vi "DG5252_VI.vi"(5 "DC Offset (0.00 V)":dbl, 6 "Frequency (1000 Hz)":dbl=1000.0, 7 "Unit (0: Vpp)":u16(ring) items=["Vpp", "Vrms", "dB"], 8 "Amplitude (1)":dbl=1.0, 9 "Waveform Function":u16(ring) items=["Sine", "Square", "Ramp", "Pulse", "Noise", "DC", "User"], 10 "Channel Selection":u16(ring) items=["Channel 1", "Channel 2"], 11 "VISA resource name":refnum<visa-resource-name>) -> ()   [LabVIEW 2017]
panel:
  out "configure error out":errorcluster
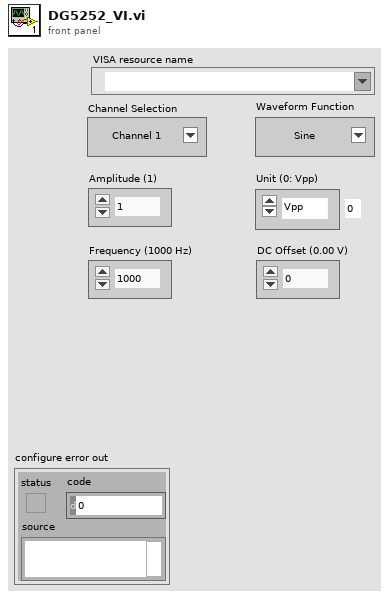
[diagram p1: front panel]
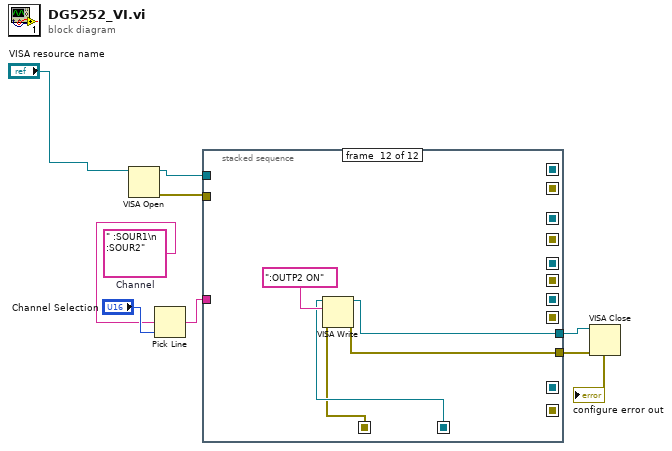
[diagram p0: block diagram]
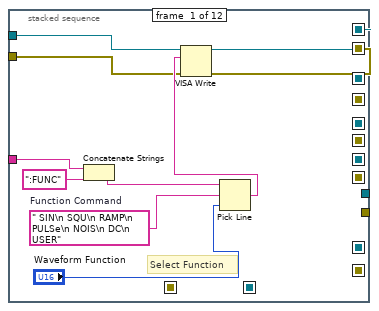
[diagram p2: hidden frame]
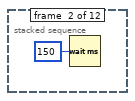
[diagram p3: hidden frame]
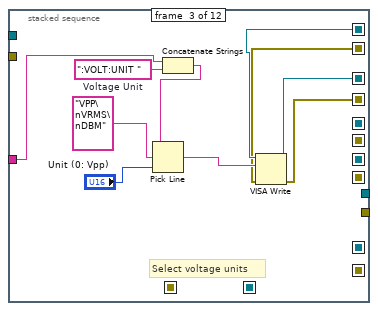
[diagram p4: hidden frame]
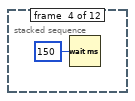
[diagram p5: hidden frame]
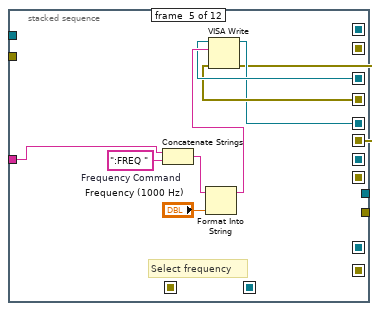
[diagram p6: hidden frame]
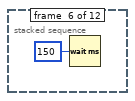
[diagram p7: hidden frame]
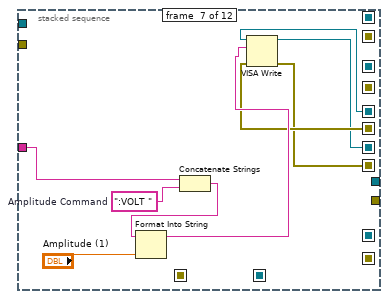
[diagram p8: hidden frame]
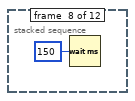
[diagram p9: hidden frame]
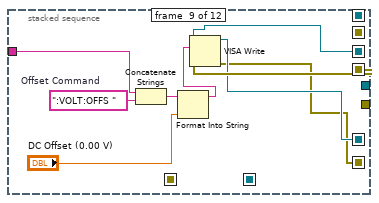
[diagram p10: hidden frame]
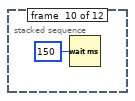
[diagram p11: hidden frame]
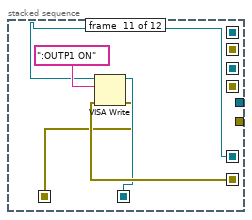
[diagram p12: hidden frame]
diagram:
  w3 = " :SOUR1\n :SOUR2"  # Channel
  n1 = VISA Open(VISA resource name="VISA resource name") -> (VISA resource name=w7:refnum<visa-resource-name>, error out=w8:errorcluster)  [unwired: 4 in]
  n2 = Pick Line(multi-line string=w3, line index="Channel Selection") -> (output string=w5:string)  [unwired: 1 in]
  n3 = stacked-sequence {
    seq-local: [w13 _ _ _ _ _ _ _ _ _ _ _] -> [_ _ w25 _ _ _ _ _ _ _ _ _]
    seq-local: [w14 _ _ _ _ _ _ _ _ _ _ _] -> [_ _ w24 _ _ _ _ _ _ _ _ _]
    seq-local: [_ _ w23 _ _ _ _ _ _ _ _ _] -> [_ _ _ _ w36 _ _ _ _ _ _ _]
    seq-local: [_ _ w22 _ _ _ _ _ _ _ _ _] -> [_ _ _ _ w35 _ _ _ _ _ _ _]
    seq-local: [_ _ _ _ w34 _ _ _ _ _ _ _] -> [_ _ _ _ _ _ w46 _ _ _ _ _]
    seq-local: [_ _ _ _ w33 _ _ _ _ _ _ _] -> [_ _ _ _ _ _ w45 _ _ _ _ _]
    seq-local: [_ _ _ _ _ _ w44 _ _ _ _ _] -> [_ _ _ _ _ _ _ _ w56 _ _ _]
    seq-local: [_ _ _ _ _ _ w43 _ _ _ _ _] -> [_ _ _ _ _ _ _ _ w55 _ _ _]
    seq-local: [_ _ _ _ _ _ _ _ w53 _ _ _] -> [_ _ _ _ _ _ _ _ _ _ w65 _]
    seq-local: [_ _ _ _ _ _ _ _ w52 _ _ _] -> [_ _ _ _ _ _ _ _ _ _ w64 _]
    seq-local: [_ _ _ _ _ _ _ _ _ _ w63 _] -> [_ _ _ _ _ _ _ _ _ _ _ w70]
    seq-local: [_ _ _ _ _ _ _ _ _ _ w62 _] -> [_ _ _ _ _ _ _ _ _ _ _ w69]
    tunnel: w7 -> [w18 _ _ _ _ _ _ _ _ _ _ _]
    tunnel: w8 -> [w17 _ _ _ _ _ _ _ _ _ _ _]
    tunnel: w5 -> [w10 _ w21 _ w32 _ w42 _ w54 _ _ _]
    tunnel: [_ _ _ _ _ _ _ _ _ _ _ w68] -> w2
    tunnel: [_ _ _ _ _ _ _ _ _ _ _ w67] -> w1
    frame #0 {
      w12 = " SIN\n SQU\n RAMP\n PULSe\n NOIS\n DC\n USER"  # Function Command
      # "Select Function"
      n4 = Concatenate Strings(w10, ":FUNC" ("string (\"\")")) -> (w15:string)
      n5 = Pick Line(string ("")=w15, multi-line string=w12, line index="Waveform Function") -> (output string=w19:string)
      n6 = VISA Write(VISA resource name=w18, write buffer=w19, error in (no error)=w17) -> (VISA resource name out=w13:refnum<visa-resource-name>, error out=w14:errorcluster)  [unwired: 1 out]
    }
    frame #1 {
      n7 = Wait (ms)(milliseconds to wait=u32 150) -> ()  [unwired: 1 out]
    }
    frame #2 {
      w27 = ":VOLT:UNIT "  # Voltage Unit
      # "Select voltage units"
      n8 = Concatenate Strings(w21, w27) -> (w26:string)
      n9 = Pick Line(string ("")=w26, multi-line string="VPP\nVRMS\nDBM", line index="Unit (0: Vpp)") -> (output string=w29:string)
      n10 = VISA Write(VISA resource name=w25, write buffer=w29, error in (no error)=w24) -> (VISA resource name out=w23:refnum<visa-resource-name>, error out=w22:errorcluster)  [unwired: 1 out]
    }
    frame #3 {
      n11 = Wait (ms)(milliseconds to wait=u32 150) -> ()  [unwired: 1 out]
    }
    frame #4 {
      w38 = ":FREQ "  # Frequency Command
      # "Select frequency"
      n12 = Concatenate Strings(w32, w38) -> (w37:string)
      n13 = Format Into String(initial string=w37, "Frequency (1000 Hz)") -> (resulting string=w40:string)  [unwired: 2 in, 1 out]
      n14 = VISA Write(VISA resource name=w36, write buffer=w40, error in (no error)=w35) -> (VISA resource name out=w34:refnum<visa-resource-name>, error out=w33:errorcluster)  [unwired: 1 out]
    }
    frame #5 {
      n15 = Wait (ms)(milliseconds to wait=u32 150) -> ()  [unwired: 1 out]
    }
    frame #6 {
      w48 = ":VOLT "  # Amplitude Command
      n16 = Concatenate Strings(w42, w48) -> (w47:string)
      n17 = Format Into String(initial string=w47, "Amplitude (1)") -> (resulting string=w50:string)  [unwired: 2 in, 1 out]
      n18 = VISA Write(VISA resource name=w46, write buffer=w50, error in (no error)=w45) -> (VISA resource name out=w44:refnum<visa-resource-name>, error out=w43:errorcluster)  [unwired: 1 out]
    }
    frame #7 {
      n19 = Wait (ms)(milliseconds to wait=u32 150) -> ()  [unwired: 1 out]
    }
    frame #8 {
      w58 = ":VOLT:OFFS "  # Offset Command
      n20 = Concatenate Strings(w54, w58) -> (w57:string)
      n21 = Format Into String(initial string=w57, "DC Offset (0.00 V)") -> (resulting string=w60:string)  [unwired: 2 in, 1 out]
      n22 = VISA Write(VISA resource name=w56, write buffer=w60, error in (no error)=w55) -> (VISA resource name out=w53:refnum<visa-resource-name>, error out=w52:errorcluster)  [unwired: 1 out]
    }
    frame #9 {
      n23 = Wait (ms)(milliseconds to wait=u32 150) -> ()  [unwired: 1 out]
    }
    frame #10 {
      n24 = VISA Write(VISA resource name=w65, write buffer=":OUTP1 ON", error in (no error)=w64) -> (VISA resource name out=w63:refnum<visa-resource-name>, error out=w62:errorcluster)  [unwired: 1 out]
    }
    frame #11 {
      n25 = VISA Write(VISA resource name=w70, write buffer=":OUTP2 ON", error in (no error)=w69) -> (VISA resource name out=w68:refnum<visa-resource-name>, error out=w67:errorcluster)  [unwired: 1 out]
    }
  }
  n26 = VISA Close(VISA resource name=w2, error in (no error)=w1) -> (error out=→"configure error out":errorcluster)
